vi "Is Canceled.vi"(8 "error in":errorcluster, 11 "measure call context in":refnum<class "Measure Call Context.lvclass">) -> (0 "error out":errorcluster, 2 "is canceled?":bool, 3 "measure call context out":refnum<class "Measure Call Context.lvclass">)   [LabVIEW 2021, in "NI Measurement Plug-In SDK.lvlib" / "Measure Call Context.lvclass"]
doc: "Returns True if the measurement has been canceled by the client. The Measurement Logic VI should poll this property and immediately return when it is True."
uses:
  Measure Call Context.lvclass
  Measure Call Context.lvclass/Measure Call Context.ctl
  <vilib>/gRPC/LabVIEW gRPC Library/grpc-lvsupport-release.lvlib
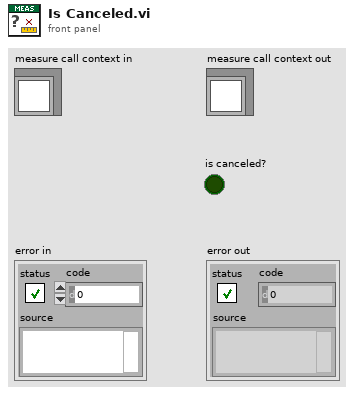
[diagram p1: front panel]
types:
  T1 = typedef "NI Measurement Plug-In SDK.lvlib/Measure Call Context.lvclass/Data.ctl" = cluster{"pin map context":T2, "gRPC ID":T3, "measurement service":refnum<class "IMeasurement Service.lvclass">, "measurement plugin service":refnum<class "Measurement Plugin Service.lvclass">, "reserved session infos":set{T4}}
  T2 = typedef "NI Measurement Plug-In SDK.lvlib/Pin Map Context.ctl" = cluster{"pin map id":string, "sites":i32[]}
  T3 = typedef "grpc-lvsupport-release.lvlib/grpcId.ctl" = u64
  T4 = typedef "ni.measurementlink.sessionmanagement.v1.api.lvlib/ni_measurementlink_sessionmanagement_v1_SessionInformation.ctl" = cluster{"session":T5, "resource_name":string, "channel_list":string, "instrument_type_id":string, "session_exists":bool, "session_reserved":bool, "channel_mappings":T6[], "annotations":T7[]}
  T5 = typedef "ni.measurementlink.sessionmanagement.v1.api.lvlib/nidevice_grpc_Session.ctl" = cluster{"name":string}
  T6 = typedef "ni.measurementlink.sessionmanagement.v1.api.lvlib/ni_measurementlink_sessionmanagement_v1_ChannelMapping.ctl" = cluster{"pin_or_relay_name":string, "site":i32, "channel":string, "multiplexer_resource_name":string, "multiplexer_route":string}
  T7 = typedef "ni.measurementlink.sessionmanagement.v1.api.lvlib/ni_measurementlink_sessionmanagement_v1_SessionInformation_AnnotationsEntry.ctl" = cluster{"key":string, "value":string}
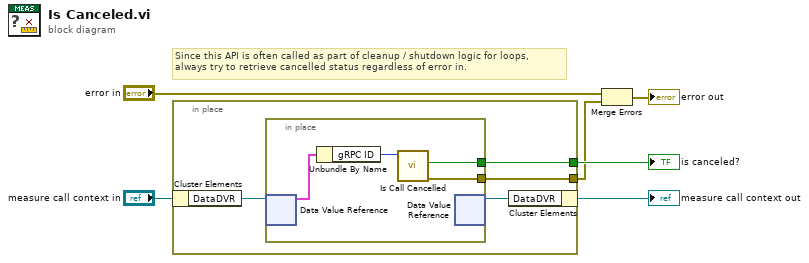
[diagram p0: block diagram]
diagram:
  # "Since this API is often called as part of cleanup / shutdown logic for loops,\nalways try to retrieve cancelled status regardless of error in."
  n1 = in-place {
    in-place-border: [w10] -> w4
    in-place-border: [w9] -> w2
    n2 = in-place-cluster #1("measure call context in") -> ("DataDVR"=w8:refnum<data-value>)
    n3 = in-place {
      in-place-border: [w14] -> w10
      in-place-border: [w13] -> w9
      n4 = in-place-dvr #2(w8) -> (w12:T1)  [unwired: 1 out]
      n5 = Unbundle By Name(w12) -> ("gRPC ID"=w11:T3)
      n6 = call <vilib>:"Is Call Cancelled.vi"("gRPCid in"=w11) -> ("error out"=w13:errorcluster, "Is Cancelled"=w14:bool)  [unwired: 8 in, 1 out]
      n7 = in-place-dvr #2() -> (w7:refnum<data-value>)  [unwired: 1 in, 1 out]
    }
    n8 = in-place-cluster #1("DataDVR"=w7) -> (→"measure call context out":refnum<class "Measure Call Context.lvclass">)
  }
  "is canceled?" <- w4
  n9 = Merge Errors("error in", w2) -> (→"error out":errorcluster)
